vi "Mechanism-read-position_RIMAS.vi"(8 "error in":errorcluster, 9 "Enable empty file warning":bool=TRUE caption="Enable", 10 "Mechanism  number":u16, 11 "Mechanism type":u16(ring) items=["Filter wheels", "Focus"]) -> (0 "error out":errorcluster, 2 "Travel (mm)  for motor steps #":dbl format="%#.3g", 3 "Position data":T1, 4 "Created/existed?":bool, 5 "Current State Position Filename out":path=path "C:/RATIR_SPM/FOCUS/Focus_postion/Focus_positions_RATIR.csv", 7 "Log file name full":path caption="Log file name")   [LabVIEW 2022 SP3]
uses:
  <vilib>/Utility/file.llb/Read From Spreadsheet File (string).vi
panel:
  out "Empty file":bool
  out "Size read":i32
  out "Mechanism name":string
  out "Read spreadsheet string":string[][](array[string])=[["Detector  ", " Axis ", " position_(mm) ", " position_steps ", " speed ", " acceleration "], ["C2 ", "1.000000", "15.000000", "0.000000", "400.000000", "4000.000000"], ["C3", "2.000000", "2.100000", "0.000000", "400.000000", "4000.000000"]]
  # "READ"
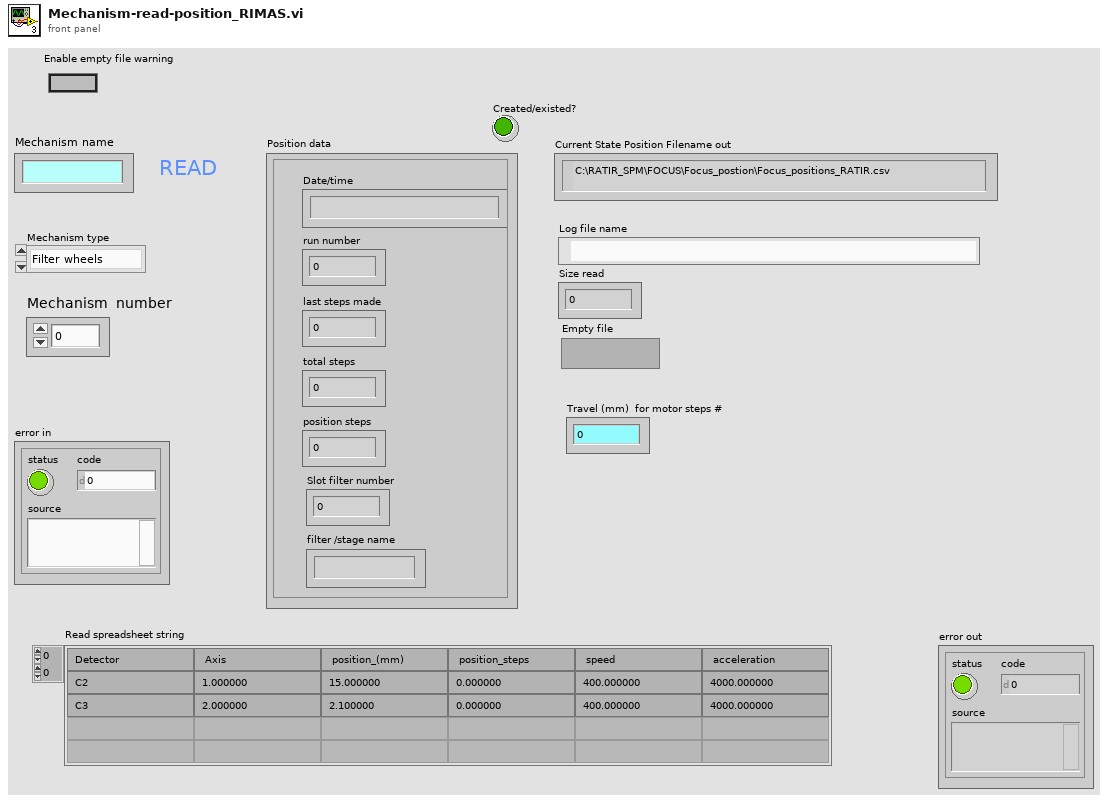
[diagram p1: front panel]
types:
  T1 = cluster{"Date/time":string, "run number":u16, "last steps made":i32, "total steps":i32, "position steps":i32, "Slot filter number":i32, "filter /stage name":string}
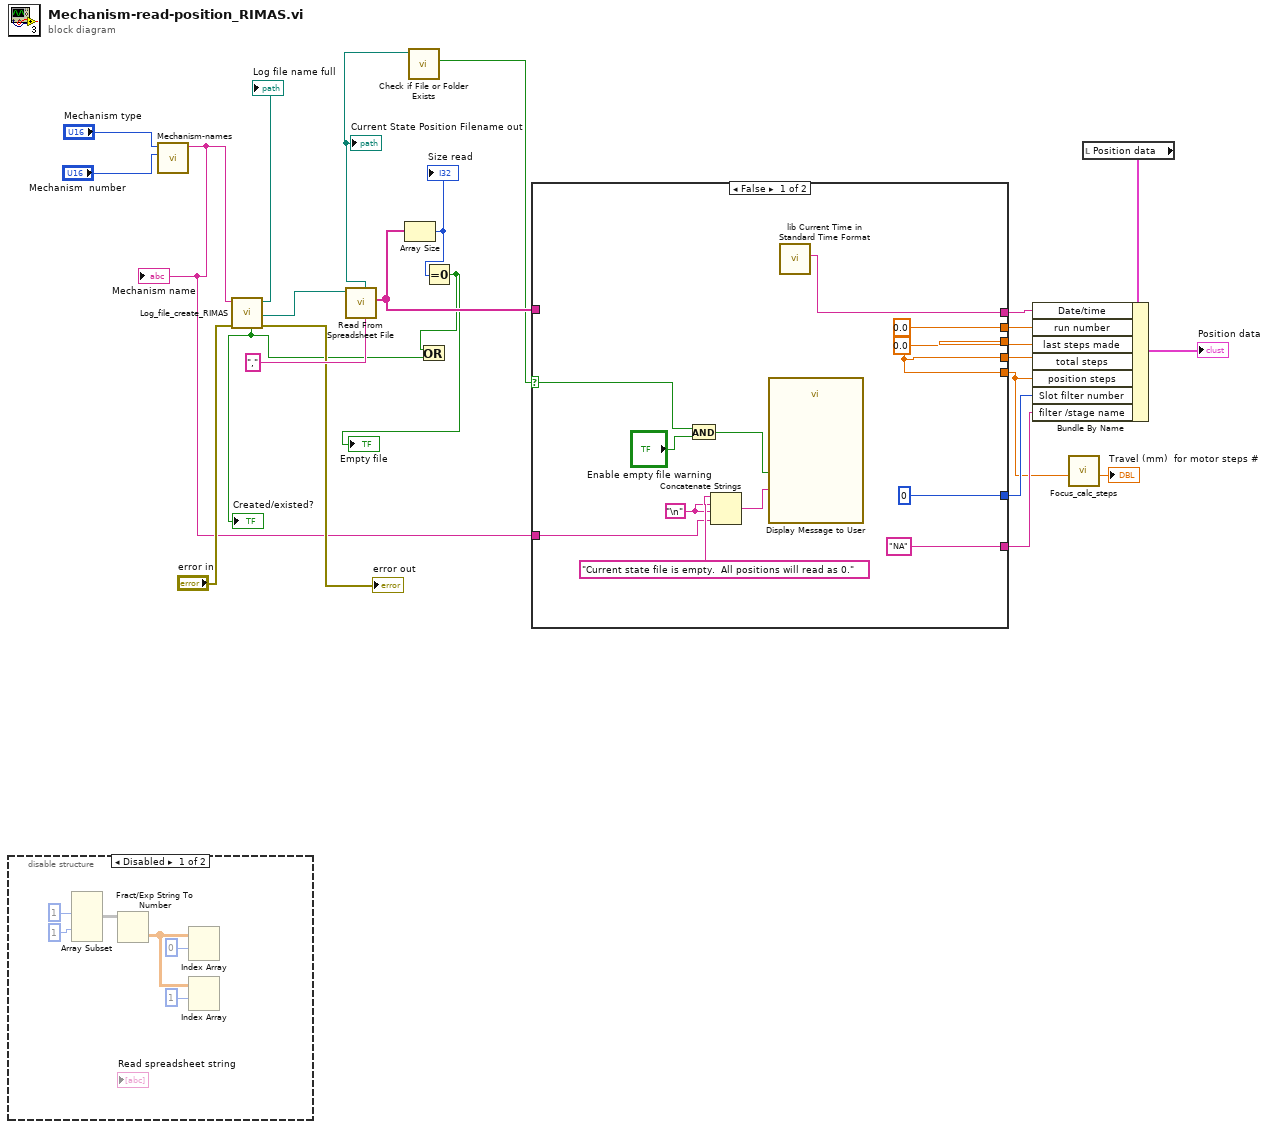
[diagram p0: block diagram]
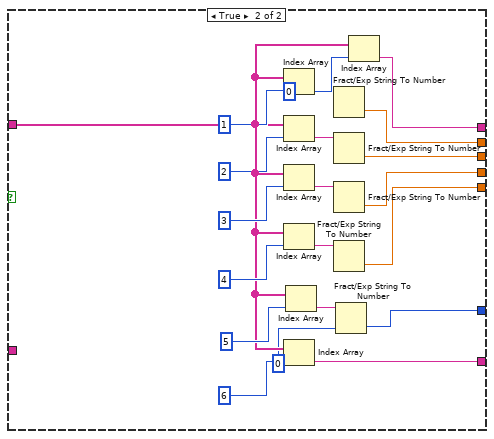
[diagram p2: hidden frame]
diagram:
  n1 = disable-structure shown="Disabled" {
    frame Disabled {
      n2 = Array Subset(index (row)=1 ("index"), index (col)=1 ("index")) -> (w30:void[][])  [unwired: 3 in]
      n3 = Fract/Exp String To Number(string=w30) -> (number=w25:dbl[][])  [unwired: 3 in, 1 out]
      n4 = Index Array(array=w25, index (row)=0) -> ()  [unwired: 1 in, 1 out]
      n5 = Index Array(array=w25, index (row)=1) -> ()  [unwired: 1 in, 1 out]
    }
    frame Enabled {
    }
  }
  n6 = call "Mechanism-names.vi"("Mechanism  number"="Mechanism  number", "Mechanism type"="Mechanism type") -> ("Mechanism name"=w3:string)  [unwired: 6 in, 3 out]
  "Mechanism name" <- w3
  n7 = call "Log_file_create_RIMAS.vi"("error in (no error)"="error in", "Mechanism name"=w3) -> ("error out"=→"error out":errorcluster, "Current state  file name full"=w17:path, "Log file name full"=→"Log file name full":path, "Created/existed?"=w10:bool)  [unwired: 4 in, 2 out]
  "Created/existed?" <- w10
  n8 = call-poly <vilib>:"Read From Spreadsheet File.vi"("delimiter (\\t)"="," ("delimiter (\\t)"), "file path (dialog if empty)"=w17) -> ("first row"=w12:string[], "new file path (Not A Path if cancelled)"=w2:path)  [unwired: 5 in, 3 out]
  "Current State Position Filename out" <- w2
  n9 = Array Size(array=w12) -> (size(s)=w11:i32)
  "Size read" <- w11
  n10 = call <vilib>:"Check if File or Folder Exists.vi"("path"=w2) -> ("file or folder exists?"=w1:bool)  [unwired: 8 in, 2 out]
  n11 = Equal To 0?(x=w11) -> (x = 0?=w9:bool)
  "Empty file" <- w9
  n12 = Or(x=w9, y=w10) -> ()  [unwired: 1 out]
  n13 = case shown="False" w1 {
    selector: w1 -> [w32 _]
    tunnel: [w42 w54] -> w21
    tunnel: [0.0 w53] -> w20
    tunnel: [w40 w52] -> w19
    tunnel: [w40 w51] -> w18
    tunnel: [w40 w50] -> w6
    tunnel: w12 -> [_ w46]
    tunnel: [0 ("offset past number") w44] -> w14
    tunnel: ["NA" ("String") w45] -> w13
    tunnel: w3 -> [w34 _]
    frame False {
      w35 = "\n"
      w40 = 0.0
      n14 = And(x=w32, y="Enable empty file warning") -> (x .and. y?=w31:bool)
      n15 = Concatenate Strings("Current state file is empty.  All positions will read as 0." ("Message"), w35, w35, w34) -> (w37:string)
      n16 = call "Display Message to User"("Enable"=w31, "Message"=w37) -> ()  [unwired: 8 in, 2 out]
      n17 = call "lib Current Time in Standard Time Format.vi"() -> ("date/time string"=w42:string)  [unwired: 11 in]
    }
    frame True {
      n18 = Index Array(array=w46, index=1) -> (element=w61:string)
      n19 = Index Array(array=w46, index=2) -> (element=w60:string)
      n20 = Index Array(array=w46, index=3) -> (element=w57:string)
      n21 = Index Array(array=w46, index=4) -> (element=w56:string)
      n22 = Index Array(array=w46, index=6) -> (element=w45:string)
      n23 = Index Array(array=w46, index=5) -> (element=w48:string)
      n24 = Fract/Exp String To Number(string=w61) -> (number=w53:dbl)  [unwired: 3 in, 1 out]
      n25 = Fract/Exp String To Number(string=w60) -> (number=w52:dbl)  [unwired: 3 in, 1 out]
      n26 = Fract/Exp String To Number(string=w57) -> (number=w51:dbl)  [unwired: 3 in, 1 out]
      n27 = Fract/Exp String To Number(string=w56) -> (number=w50:dbl)  [unwired: 3 in, 1 out]
      n28 = Fract/Exp String To Number(string=w48, default (0 dbl)=0 ("default (0 DBL)")) -> (number=w44:i32)  [unwired: 2 in, 1 out]
      n29 = Index Array(array=w46, index=0) -> (element=w54:string)
    }
  }
  n30 = call "Focus_calc_steps.vi"("Motor steps #"=w6) -> ("Travel (mm)  for motor steps #"=→"Travel (mm)  for motor steps #":dbl)  [unwired: 9 in, 1 out]
  n31 = local read "Position data"() -> (w23:T1)
  n32 = Bundle By Name(cluster=w23, "Date/time"=w21, "run number"=w20, "last steps made"=w19, "total steps"=w18, "position steps"=w6, "Slot filter number"=w14, "filter /stage name"=w13) -> (→"Position data":T1)
